vi "CorrLast2Img.vi"() -> ()   [LabVIEW 2014]
uses:
  <vilib>/Analysis/2dsp.llb/2D Cross Correlation (DBL).vi
  <userlib>/Nanonis Prog Interface V5/Nanonis Prog Interface.lvlib
  <vilib>/Analysis/NI_AALPro.lvlib
panel:
  out "Correl 2":picture
  out "Y drift 2nd corr":i32
  out "X drift 2nd corr":i32
  in  "Direction (clockwise)":T1(ring)
  in  "method":T2(ring)
  out "Correl":picture
  out "pixel":i32=256
  out "Y drift":i32
  out "X drift":i32
  in  "First":i32=5 min=1 max=26
  in  "stop":bool
  in  "second":i32=4 min=0 max=26
  out "element 2":cluster{"last mod":timestamp, "path out":path}={"last mod"=timestamp(3554755212 s since 1904-01-01), "path out"=path "D:/STM Data/082016/160823_095600_2mol_chain/topo/160823_10-00-11_SPM001.sxm"}
  out "element":cluster{"last mod":timestamp, "path out":path}={"last mod"=timestamp(3554755074 s since 1904-01-01), "path out"=path "D:/STM Data/082016/160823_095600_2mol_chain/topo/160823_09-57-54_SPM001.sxm"}
  out "x-y":i32[](array[numeric])
  out "Img1 2":picture
  out "Img1":picture
  in  "Read channel 2":i8 min=-1
  in  "Path":path=path "D:/STM Data/082016/160823_095600_2mol_chain/topo"
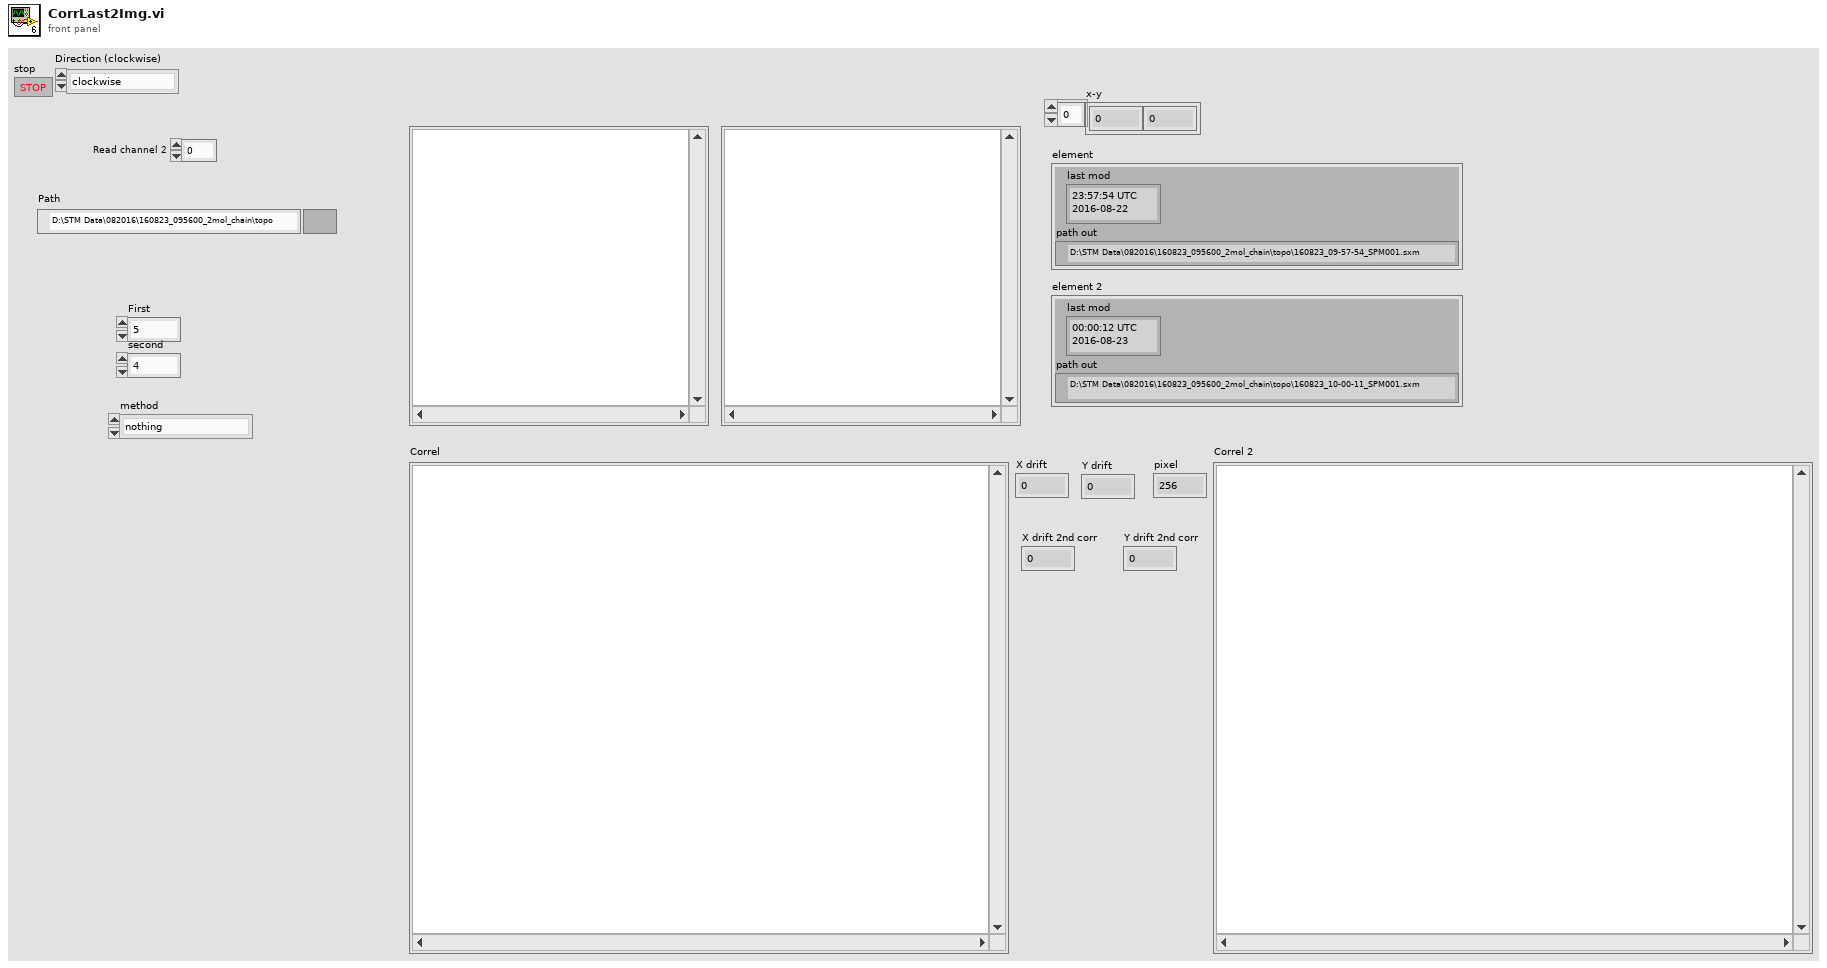
[diagram p1: front panel]
types:
  T1 = enum16{"clockwise", "counter-clockwise", "nothing"}
  T2 = enum16{"nothing", "average", "8bit", "average/plane", "minimum", "plane", "average/stddev", "plane/average"}
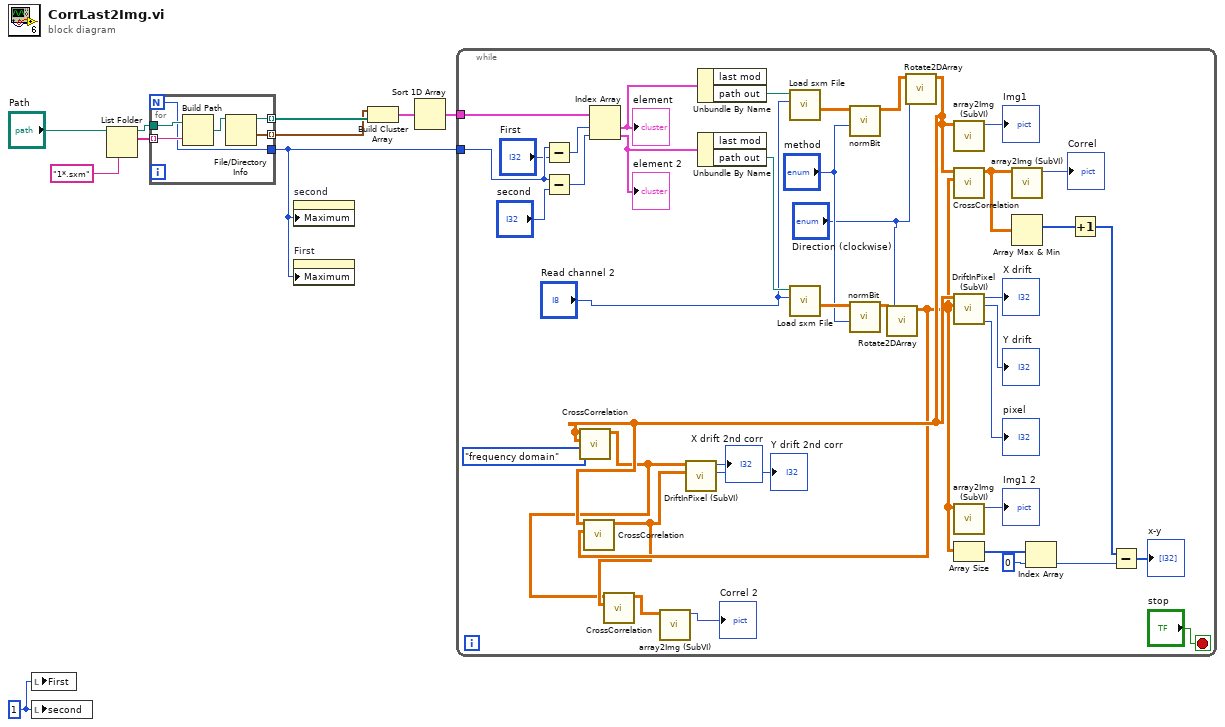
[diagram p0: block diagram]
diagram:
  w1 = 1 ("second")
  n1 = local write "First"(w1) -> ()
  n2 = local write "second"(w1) -> ()
  n3 = List Folder(path="Path", pattern="1*.sxm") -> (path out=w8:path, filenames=w9:string[])  [unwired: 2 in, 2 out]
  n4 = for {
    N -> [w11]
    tunnel: w9 -> [w16] mode=indexing
    tunnel: w8 -> [w15]
    tunnel: [w13] -> w5 mode=indexing
    tunnel: [w12] -> w6 mode=indexing
    tunnel: [w11] -> w2
    n5 = Build Path(base path=w15, name or relative path=w16) -> (appended path=w14:path)
    n6 = File/Directory Info(path=w14) -> (path out=w12:path, last mod=w13:timestamp)  [unwired: 1 in, 5 out]
  }
  n7 = property on="second" class="DigNum (strict)"("Maximum"=w2) -> ()  [unwired: 2 in, 2 out]
  n8 = property on="First" class="DigNum (strict)"("Maximum"=w2) -> ()  [unwired: 2 in, 2 out]
  n9 = Build Cluster Array(w5, w6) -> (w4:cluster{"last mod":timestamp, "path out":path}[])
  n10 = Sort 1D Array(array=w4) -> (sorted array=w3:cluster{"last mod":timestamp, "path out":path}[])
  n11 = while {
    tunnel: w3 -> [w48]
    tunnel: w2 -> [w41]
    stop <- "stop" stop-if-true
    n12 = Subtract(x=w41, y="First") -> (x-y=w43:i32)
    n13 = Subtract(x=w41, y="second") -> (x-y=w42:i32)
    n14 = Index Array(array=w48, index #1=w43, index #2=w42) -> (element #1=w47:cluster{"last mod":timestamp, "path out":path}, element #2=w45:cluster{"last mod":timestamp, "path out":path})
    "element" <- w47
    "element 2" <- w45
    n15 = Unbundle By Name(w47) -> ("path out"=w46:path)  [unwired: 1 out]
    n16 = Unbundle By Name(w45) -> ("path out"=w44:path)  [unwired: 1 out]
    n17 = call <userlib>:"Load sxm File.vi"("Read channel"="Read channel 2", "Scan data file"=w46) -> ("Data"=w37:sgl[][])  [unwired: 4 in, 5 out]
    n18 = call <userlib>:"Load sxm File.vi"("Read channel"="Read channel 2", "Scan data file"=w44) -> ("Data"=w36:sgl[][])  [unwired: 4 in, 5 out]
    n19 = call "normBit.vi"("method"="method", "Rxy"=w37) -> ("Array"=w29:dbl[][])  [unwired: 8 in, 1 out]
    n20 = call "normBit.vi"("method"="method", "Rxy"=w36) -> ("Array"=w28:dbl[][])  [unwired: 8 in, 1 out]
    n21 = call "Rotate2DArray.vi"("Direction (clockwise)"="Direction (clockwise)", "Array in"=w28) -> ("Array Out"=w24:dbl[][])  [unwired: 9 in]
    n22 = call "Rotate2DArray.vi"("Direction (clockwise)"="Direction (clockwise)", "Array in"=w29) -> ("Array Out"=w25:dbl[][])  [unwired: 9 in]
    n23 = call-poly <vilib>:"CrossCorrelation.vi"("algorithm"=enum32{"direct", "frequency domain"}."frequency domain", "Y"=w25, "X"=w25) -> ("Rxy"=w20:dbl[][])  [unwired: 7 in, 1 out]
    n24 = call-poly <vilib>:"CrossCorrelation.vi"("Y"=w24, "X"=w25) -> ("Rxy"=w21:dbl[][])  [unwired: 8 in, 1 out]
    n25 = call-poly <vilib>:"CrossCorrelation.vi"("Y"=w21, "X"=w20) -> ("Rxy"=w19:dbl[][])  [unwired: 8 in, 1 out]
    n26 = call "array2Img (SubVI).vi"("Rxy"=w19) -> ("new picture"=→"Correl 2":picture)  [unwired: 10 in]
    n27 = call "DriftInPixel (SubVI).vi"("New image"=w21, "Ref image"=w20) -> ("Y drift"=→"Y drift 2nd corr":i32, "X drift"=→"X drift 2nd corr":i32)  [unwired: 7 in, 1 out]
    n28 = call "array2Img (SubVI).vi"("Rxy"=w25) -> ("new picture"=→"Img1":picture)  [unwired: 10 in]
    n29 = call-poly <vilib>:"CrossCorrelation.vi"("Y"=w24, "X"=w25) -> ("Rxy"=w32:dbl[][])  [unwired: 8 in, 1 out]
    n30 = call "DriftInPixel (SubVI).vi"("New image"=w24, "Ref image"=w25) -> ("pixel"=→"pixel":i32, "Y drift"=→"Y drift":i32, "X drift"=→"X drift":i32)  [unwired: 7 in]
    n31 = call "array2Img (SubVI).vi"("Rxy"=w24) -> ("new picture"=→"Img1 2":picture)  [unwired: 10 in]
    n32 = Array Size(array=w24) -> (size(s)=w53:i32[])
    n33 = call "array2Img (SubVI).vi"("Rxy"=w32) -> ("new picture"=→"Correl":picture)  [unwired: 10 in]
    n34 = Array Max & Min(array=w32) -> (max index (indices)=w54:i32[])  [unwired: 3 out]
    n35 = Index Array(array=w53, index=0) -> (element=w51:i32)
    n36 = Increment(x=w54) -> (x+1=w50:i32[])
    n37 = Subtract(x=w50, y=w51) -> (x-y=→"x-y":i32[])
  }
